vi "dual_color_3D_continuous_scan_with_delay_and_ETL_control.vi"() -> ()   [LabVIEW 2017]
uses:
  <vilib>/DAQmx/write.llb/DAQmx Write (Analog DBL 1Chan 1Samp).vi
  <vilib>/DAQmx/write.llb/DAQmx Write (Analog 1D DBL NChan 1Samp).vi
  <vilib>/DAQmx/write.llb/DAQmx Write (Analog 2D DBL NChan NSamp).vi
  <vilib>/DAQmx/create/channels.llb/DAQmx Create Channel (AO-Voltage-Basic).vi
  <vilib>/DAQmx/miscellaneous.llb/DAQmx Fill In Error Info.vi
  <vilib>/Utility/file.llb/Read Delimited Spreadsheet (DBL).vi
  <vilib>/measure/mascope.llb/Transition Measurements 1 chan.vi
  <vilib>/DAQmx/configure/timing.llb/DAQmx Timing (Sample Clock).vi
  <vilib>/DAQmx/configure/trigger.llb/DAQmx Start Trigger (Digital Edge).vi
  <vilib>/DAQmx/configure/trigger.llb/DAQmx Start Trigger (None).vi
  <vilib>/measure/NI_MAPro.lvlib
panel:
  in  "Listbox 2":i32(listbox)=3
  in  "Listbox":i32(listbox)=1
  in  "ETL voltage offset":dbl(slide) min=-10.0 max=10.0 step=0.05 scale=-10.0..10.0
  out "mirx raw 2":dbl[](array[numeric])
  out "Delay":dbl
  out "Sampling rate":i32
  out "ETL3":waveform(dbl)(graph)
  out "mirror y":waveform(dbl)(graph)
  out "mirror x":waveform(dbl)(graph)
  out "Laser2":waveform(dbl)(graph)
  out "Laser1":waveform(dbl)(graph)
  out "camera":waveform(dbl)(graph)
  out "mirx transition duration":dbl
  out "transition duration":dbl
  out "etl3 timing array":dbl[](array[numeric])
  out "mirror y timing array":dbl[](array[numeric])
  out "mirror x timing array":dbl[](array[numeric])
  out "Laser2 timing array":dbl[](array[numeric])
  out "Laser1 timing array":dbl[](array[numeric])
  out "camera timing array":dbl[](array[numeric])
  out "etl raw":dbl[](array[numeric])
  out "miry raw":dbl[](array[numeric])
  out "mirx raw":dbl[](array[numeric])
  out "Laser2 Intensity":dbl
  out "Laser1 Intensity":dbl
  out "Off Time":dbl
  out "On Time":dbl
  out "Number of slices":dbl
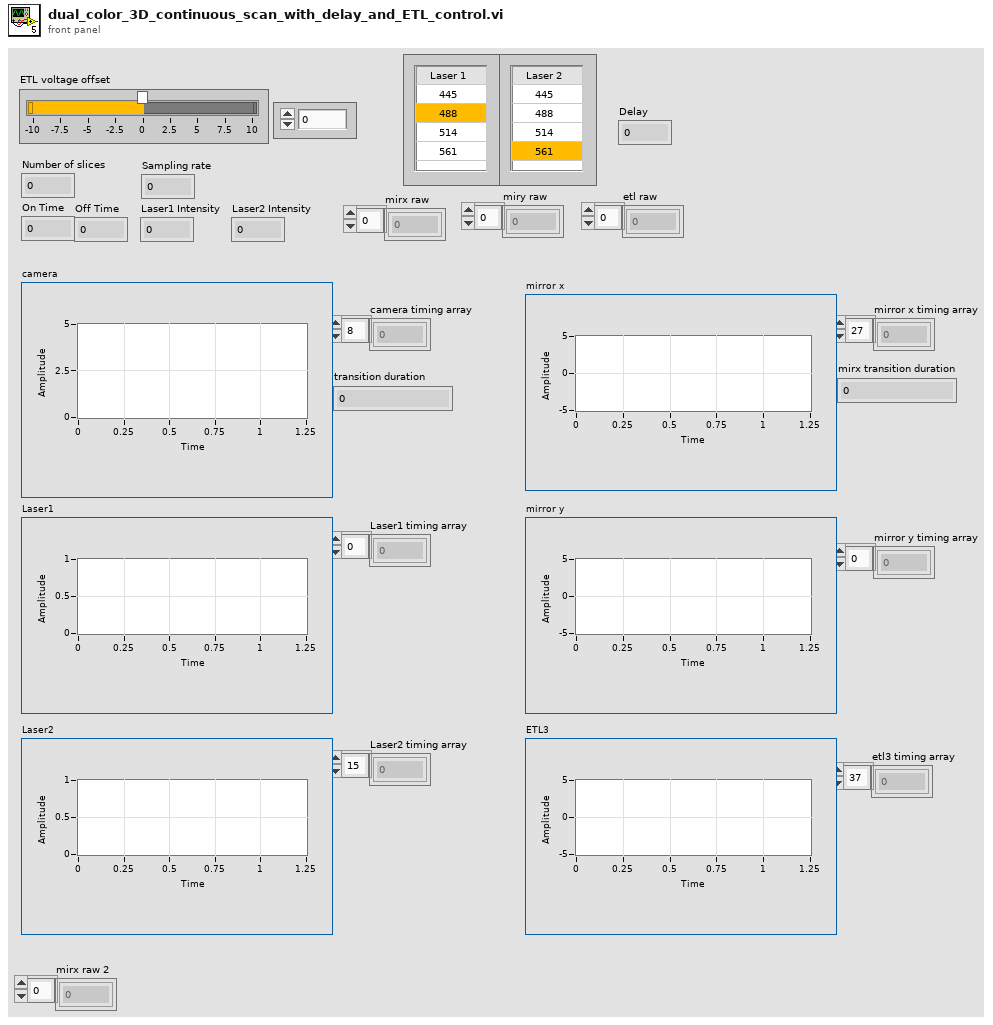
[diagram p1: front panel]
types:
  T1 = enum32{"Invalid", "Standard", "Closed", "Hidden", "Minimized", "Maximized"}
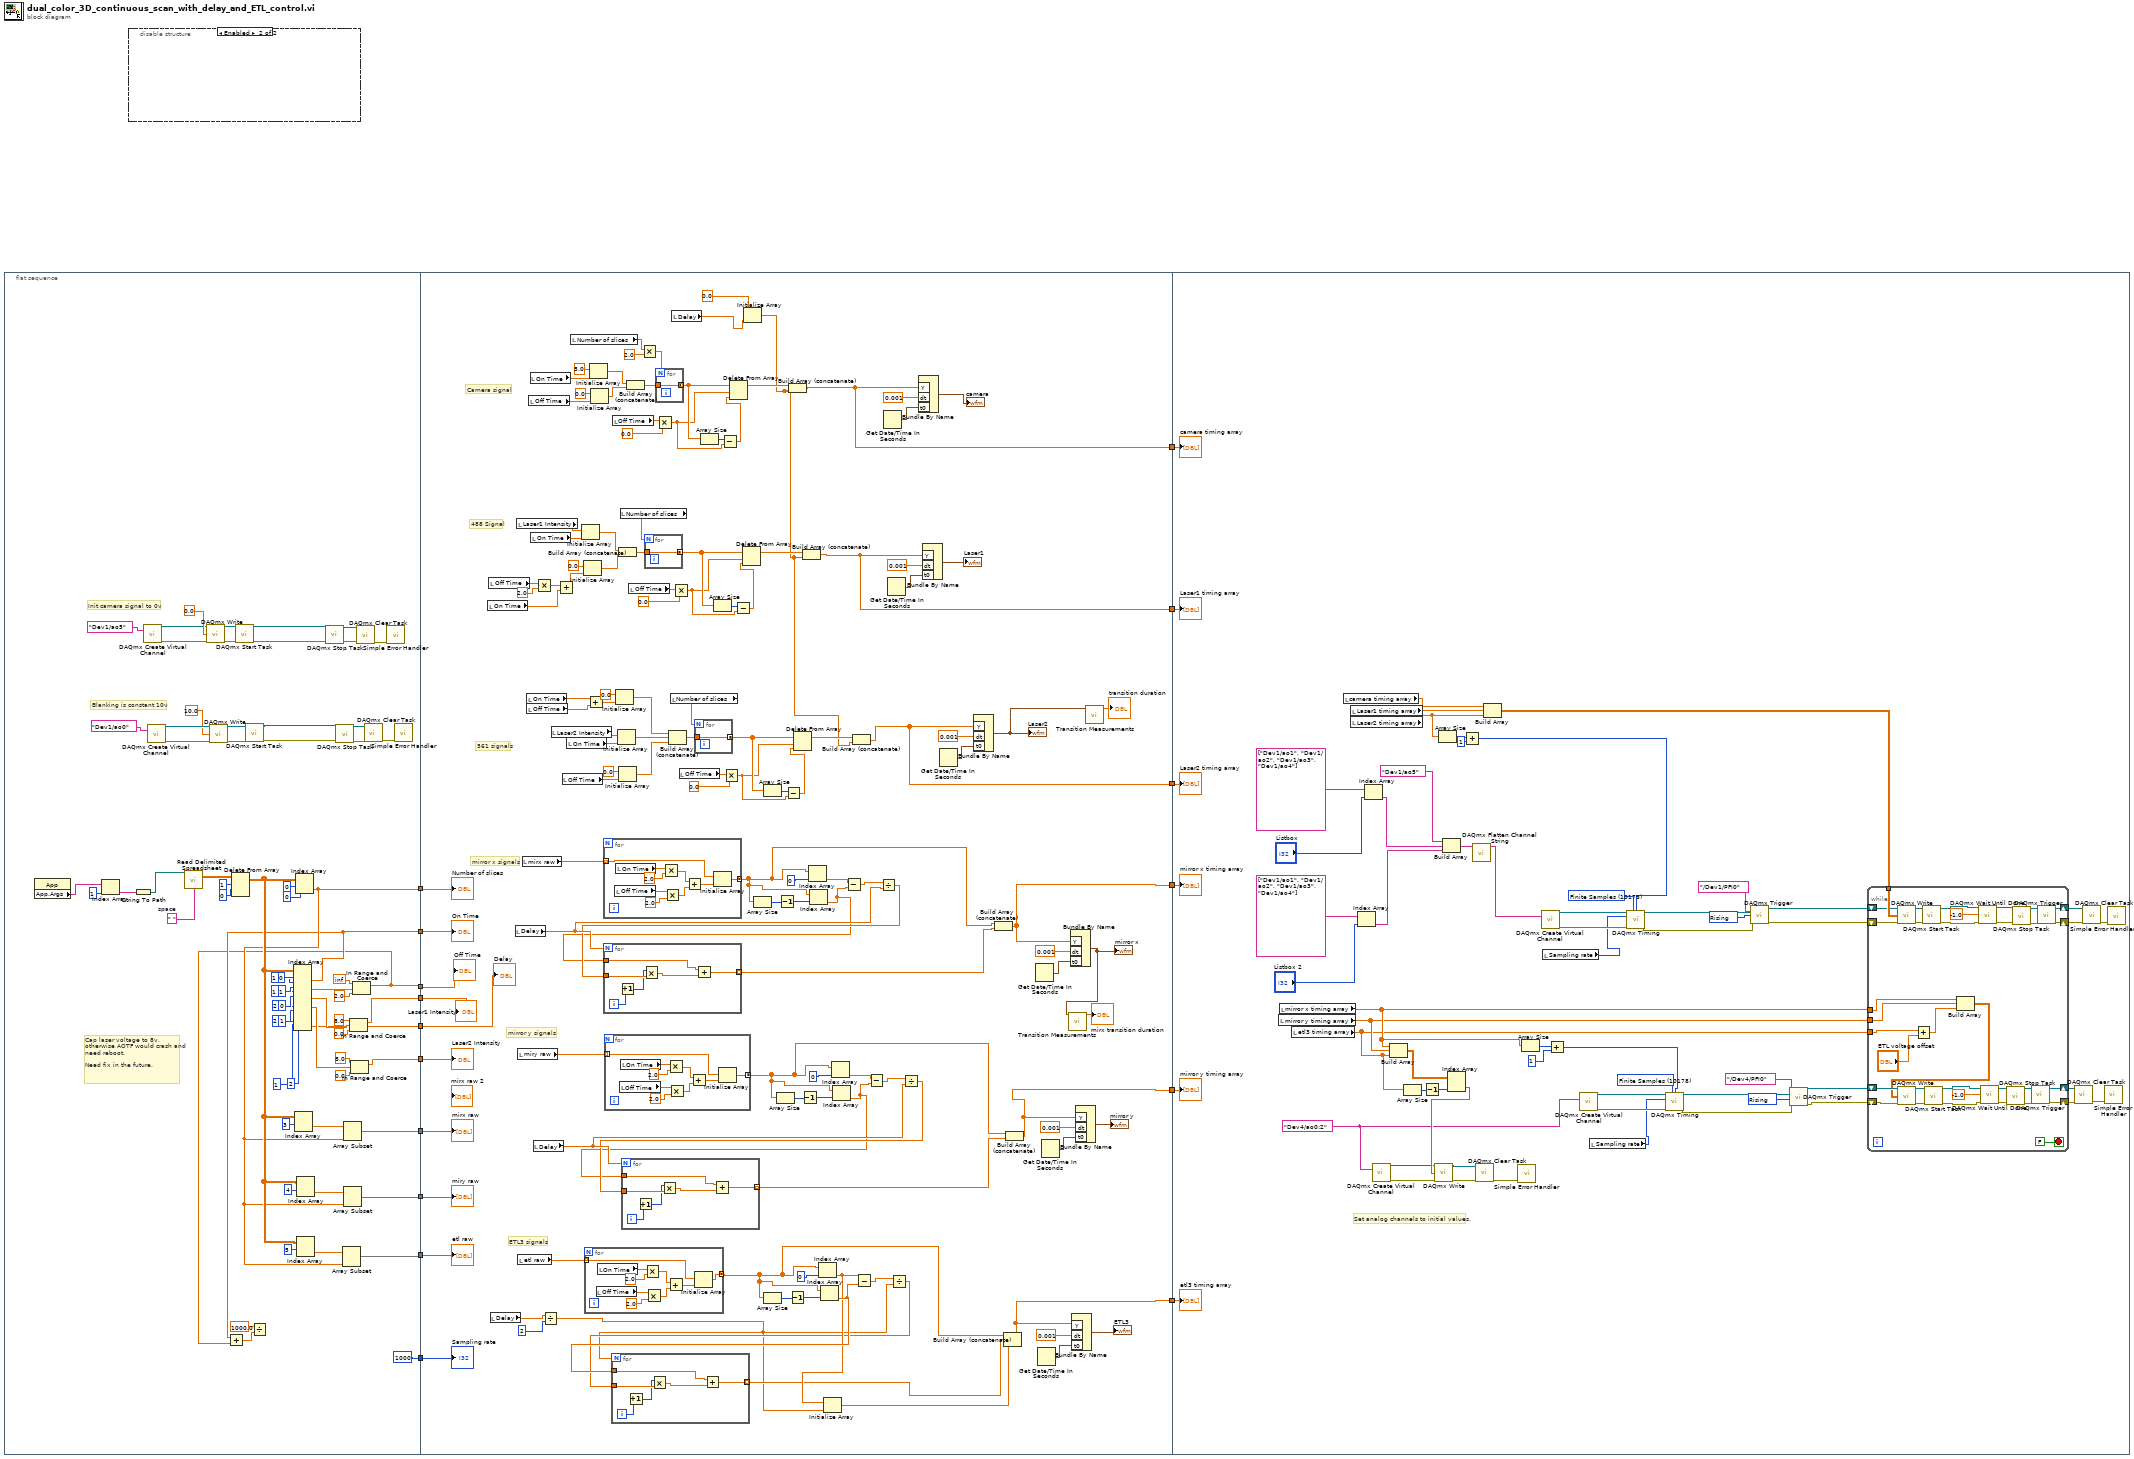
[diagram p0: block diagram]
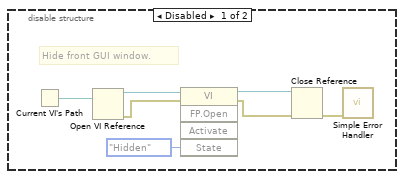
[diagram p2: hidden frame]
diagram:
  n1 = flat-sequence {
    tunnel: [w62] -> w16
    tunnel: [w48] -> w15
    tunnel: [w47] -> w14
    tunnel: [w39] -> w13
    tunnel: [w37] -> w12
    tunnel: [w61] -> w11
    tunnel: [w60] -> w10
    tunnel: [w59] -> w9
    tunnel: [1000] -> w2
    tunnel: [w34] -> w1
    tunnel: w16 -> [w146]
    tunnel: w15 -> [w145]
    tunnel: w14 -> [w144]
    tunnel: w13 -> [w143]
    tunnel: w12 -> [w142]
    tunnel: w11 -> [w141]
    tunnel: w10 -> [w140]
    tunnel: w9 -> [w139]
    tunnel: [w138] -> w8
    tunnel: [w137] -> w7
    tunnel: [w136] -> w6
    tunnel: [w135] -> w5
    tunnel: [w125] -> w4
    tunnel: [w124] -> w3
    tunnel: w2 -> [w126]
    tunnel: w1 -> [w122]
    tunnel: w8 -> [w300]
    tunnel: w7 -> [w299]
    tunnel: w6 -> [w298]
    tunnel: w5 -> [w297]
    tunnel: w4 -> [w296]
    tunnel: w3 -> [w295]
    frame #0 {
      w63 = " "  # space
      # "Init camera signal to 0v"
      # "Cap laser voltage to 8v, otherwise AOTF would crash and need reboot. \n\nNeed fix in the future."
      # "Blanking is constant 10v"
      n2 = property class="App"() -> ("App.Args"=w51:string[])  [unwired: 2 in, 2 out]
      n3 = Index Array(array=w51, index=1) -> (element=w50:string)
      n4 = String To Path(string=w50) -> (path=w49:path)
      n5 = call-poly <vilib>:"DAQmx Create Virtual Channel.vi"("physical channels"=tag "Dev1/ao5") -> ("task out"=w20:refnum<k21>, "error out"=w19:errorcluster)  [unwired: 13 in]
      n6 = call-poly <vilib>:"DAQmx Create Virtual Channel.vi"("physical channels"=tag "Dev1/ao0") -> ("task out"=w57:refnum<k21>, "error out"=w58:errorcluster)  [unwired: 13 in]
      n7 = call-poly <vilib>:"Read Delimited Spreadsheet.vi"("file path (dialog if empty)"=w49, "delimiter (\\t)"=w63) -> ("all rows"=w81:dbl[][])  [unwired: 8 in, 5 out]
      n8 = call-poly <vilib>:"DAQmx Write.vi"("task/channels in"=w20, "data"=0.0, "error in"=w19) -> ("task out"=w27:refnum<k21>, "error out"=w26:errorcluster)  [unwired: 10 in, 1 out]
      n9 = call-poly <vilib>:"DAQmx Write.vi"("task/channels in"=w57, "data"=10.0, "error in"=w58) -> ("task out"=w33:refnum<k21>, "error out"=w32:errorcluster)  [unwired: 10 in, 1 out]
      n10 = Delete From Array(array=w81, length=1, index (row)=0) -> (array with subset deleted=w82:dbl[][])  [unwired: 1 in, 1 out]
      n11 = call <vilib>:"DAQmx Start Task.vi"("task/channels in"=w27, "error in"=w26) -> ("task out"=w18:refnum<k21>, "error out"=w17:errorcluster)  [unwired: 12 in]
      n12 = call <vilib>:"DAQmx Start Task.vi"("task/channels in"=w33, "error in"=w32) -> ("task out"=w29:refnum<k21>, "error out"=w28:errorcluster)  [unwired: 12 in]
      n13 = Index Array(array=w82, index (row) #1=1 ("index (row)"), index (col) #1=0 ("disabled index (col)"), index (row) #2=1 ("index (row)"), index (col) #2=1 ("disabled index (col)"), index (row) #3=2 ("index (row)"), index (col) #3=0 ("disabled index (col)"), index (row) #4=2 ("index (row)"), index (col) #4=1 ("disabled index (col)"), index (row) #6=1 ("index (row)"), index (col) #6=2 ("disabled index (col)")) -> (element #1=w48:dbl, element #2=w86:dbl, element #3=w40:dbl, element #4=w38:dbl, element #6=w34:dbl)  [unwired: 2 in, 1 out]
      n14 = Index Array(array=w82, index (row)=3) -> (element=w83:dbl[])  [unwired: 1 in]
      n15 = Index Array(array=w82, index (row)=0, index (col)=0 ("disabled index (col)")) -> (element=w62:dbl)
      n16 = Index Array(array=w82, index (row)=5) -> (element=w85:dbl[])  [unwired: 1 in]
      n17 = Index Array(array=w82, index (row)=4) -> (element=w84:dbl[])  [unwired: 1 in]
      n18 = call <vilib>:"DAQmx Stop Task.vi"("task/channels in"=w18, "error in"=w17) -> ("task out"=w24:refnum<k21>, "error out"=w25:errorcluster)  [unwired: 12 in]
      n19 = call <vilib>:"DAQmx Stop Task.vi"("task/channels in"=w29, "error in"=w28) -> ("task out"=w31:refnum<k21>, "error out"=w30:errorcluster)  [unwired: 12 in]
      n20 = Array Subset(array=w85, length=w62) -> (w59:dbl[])  [unwired: 1 in]
      n21 = Array Subset(array=w83, length=w62) -> (w61:dbl[])  [unwired: 1 in]
      n22 = Array Subset(array=w84, length=w62) -> (w60:dbl[])  [unwired: 1 in]
      n23 = In Range and Coerce(upper limit=8.0, x=w40, lower limit=0.0) -> (coerced(x)=w39:dbl)  [unwired: 1 out]
      n24 = In Range and Coerce(upper limit=8.0, x=w38, lower limit=0.0) -> (coerced(x)=w37:dbl)  [unwired: 1 out]
      n25 = In Range and Coerce(upper limit=inf, x=w86, lower limit=2.0) -> (coerced(x)=w47:dbl)  [unwired: 1 out]
      n26 = Add(x=w48, y=w47) -> (x+y=w45:dbl)
      n27 = Divide(x=1000.0, y=w45) -> ()  [unwired: 1 out]
      n28 = call <vilib>:"DAQmx Clear Task.vi"("task in"=w24, "error in"=w25) -> ("error out"=w21:errorcluster)  [unwired: 13 in]
      n29 = call <vilib>:"DAQmx Clear Task.vi"("task in"=w31, "error in"=w30) -> ("error out"=w56:errorcluster)  [unwired: 13 in]
      n30 = call <vilib>:"Simple Error Handler.vi"("error in (no error)"=w21) -> ()  [unwired: 4 in, 5 out]
      n31 = call <vilib>:"Simple Error Handler.vi"("error in (no error)"=w56) -> ()  [unwired: 4 in, 5 out]
    }
    frame #1 {
      # "ETL3 signals"
      # "mirror y signals"
      # "mirror x signals"
      # "561 signals"
      # "488 Signal"
      # "Camera signal"
      n32 = local read "On Time"() -> (w193:dbl)
      n33 = local read "Off Time"() -> (w196:dbl)
      n34 = local read "Delay"() -> (w92:dbl)
      n35 = local read "Delay"() -> (w113:dbl)
      n36 = local read "Laser1 Intensity"() -> (w200:dbl)
      n37 = local read "miry raw"() -> (w160:dbl[])
      n38 = local read "etl raw"() -> (w159:dbl[])
      n39 = local read "mirx raw"() -> (w161:dbl[])
      n40 = local read "On Time"() -> (w167:dbl)
      n41 = local read "Off Time"() -> (w178:dbl)
      n42 = local read "Off Time"() -> (w215:dbl)
      n43 = local read "On Time"() -> (w216:dbl)
      n44 = local read "On Time"() -> (w199:dbl)
      n45 = local read "Delay"() -> (w103:dbl)
      n46 = Multiply(x=w196, y=2.0) -> (x*y=w194:dbl)
      n47 = Divide(x=w92, y=2 ("index")) -> (x/y=w87:dbl)
      n48 = local read "Laser2 Intensity"() -> (w181:dbl)
      n49 = Add(x=w194, y=w193) -> (x+y=w192:dbl)
      n50 = local read "Off Time"() -> (w163:dbl)
      n51 = local read "On Time"() -> (w180:dbl)
      n52 = local read "Number of slices"() -> (w208:dbl)
      n53 = Initialize Array(w200, w199) -> (w198:dbl[])
      n54 = Initialize Array(0.0 ("element"), w192) -> (w191:dbl[])
      n55 = for {
        tunnel: w159 -> [w231] mode=indexing
        tunnel: [w230] -> w95 mode=concatenating
        n56 = local read "Off Time"() -> (w236:dbl)
        n57 = local read "On Time"() -> (w234:dbl)
        n58 = Multiply(x=w234, y=2.0) -> (x*y=w235:dbl)
        n59 = Multiply(x=w236, y=2.0) -> (x*y=w237:dbl)
        n60 = Add(x=w235, y=w237) -> (x+y=w238:dbl)
        n61 = Initialize Array(w231, w238) -> (w230:dbl[])
      }
      n62 = Add(x=w167, y=w178) -> (x+y=w177:dbl)
      n63 = Initialize Array(5.0 ("element"), w216) -> (w213:dbl[])
      n64 = Initialize Array(0.0 ("element"), w215) -> (w212:dbl[])
      n65 = for {
        tunnel: w161 -> [w255] mode=indexing
        tunnel: [w254] -> w116 mode=concatenating
        n66 = local read "Off Time"() -> (w260:dbl)
        n67 = local read "On Time"() -> (w262:dbl)
        n68 = Multiply(x=w262, y=2.0) -> (x*y=w261:dbl)
        n69 = Multiply(x=w260, y=2.0) -> (x*y=w259:dbl)
        n70 = Add(x=w261, y=w259) -> (x+y=w258:dbl)
        n71 = Initialize Array(w255, w258) -> (w254:dbl[])
      }
      n72 = for {
        tunnel: w160 -> [w240] mode=indexing
        tunnel: [w239] -> w104 mode=concatenating
        n73 = local read "Off Time"() -> (w245:dbl)
        n74 = local read "On Time"() -> (w243:dbl)
        n75 = Multiply(x=w243, y=2.0) -> (x*y=w244:dbl)
        n76 = Multiply(x=w245, y=2.0) -> (x*y=w246:dbl)
        n77 = Add(x=w244, y=w246) -> (x+y=w247:dbl)
        n78 = Initialize Array(w240, w247) -> (w239:dbl[])
      }
      n79 = local read "Off Time"() -> (w207:dbl)
      n80 = Initialize Array(0.0 ("element"), w177) -> (w166:dbl[])
      n81 = Initialize Array(w181, w180) -> (w165:dbl[])
      n82 = Initialize Array(0.0 ("element"), w163) -> (w162:dbl[])
      n83 = Build Array (concatenate)(w198, w191) -> (w189:dbl[])
      n84 = local read "Number of slices"() -> (w190:dbl)
      n85 = Build Array (concatenate)(w213, w212) -> (w211:dbl[])
      n86 = local read "Off Time"() -> (w185:dbl)
      n87 = Multiply(x=w208, y=2.0) -> (x*y=w210:dbl)
      n88 = for {
        N: w190 -> [_]
        tunnel: w189 -> [w264]
        tunnel: [w264] -> w186 mode=concatenating
      }
      n89 = for {
        N: w210 -> [_]
        tunnel: w211 -> [w265]
        tunnel: [w265] -> w205 mode=concatenating
      }
      n90 = Multiply(x=w207, y=0.0) -> (x*y=w203:dbl)
      n91 = Build Array (concatenate)(w166, w165, w162) -> (w175:dbl[])
      n92 = local read "Number of slices"() -> (w176:dbl)
      n93 = local read "Delay"() -> (w121:dbl)
      n94 = Multiply(x=w185, y=0.0) -> (x*y=w183:dbl)
      n95 = local read "Off Time"() -> (w171:dbl)
      n96 = for {
        N: w176 -> [_]
        tunnel: w175 -> [w263]
        tunnel: [w263] -> w172 mode=concatenating
      }
      n97 = Array Size(array=w205) -> (size(s)=w204:i32)
      n98 = Array Size(array=w186) -> (size(s)=w188:i32)
      n99 = Subtract(x=w204, y=w203) -> (x-y=w202:dbl)
      n100 = Multiply(x=w171, y=0.0) -> (x*y=w169:dbl)
      n101 = Delete From Array(array=w205, length=w203, index=w202) -> (array with subset deleted=w201:dbl[])  [unwired: 1 out]
      n102 = Subtract(x=w188, y=w183) -> (x-y=w187:dbl)
      n103 = Delete From Array(array=w186, length=w183, index=w187) -> (array with subset deleted=w182:dbl[])  [unwired: 1 out]
      n104 = Initialize Array(0.0 ("y"), w121) -> (w120:dbl[])
      n105 = Array Size(array=w116) -> (size(s)=w117:i32)
      n106 = Array Size(array=w172) -> (size(s)=w174:i32)
      n107 = Array Size(array=w95) -> (size(s)=w98:i32)
      n108 = Array Size(array=w104) -> (size(s)=w107:i32)
      n109 = Decrement(x=w117) -> (x-1=w115:i32)
      n110 = Subtract(x=w174, y=w169) -> (x-y=w173:dbl)
      n111 = Build Array (concatenate)(w201, w120) -> (w138:dbl[])
      n112 = Decrement(x=w98) -> (x-1=w97:i32)
      n113 = Delete From Array(array=w172, length=w169, index=w173) -> (array with subset deleted=w168:dbl[])  [unwired: 1 out]
      n114 = Decrement(x=w107) -> (x-1=w106:i32)
      n115 = Build Array (concatenate)(w182, w120) -> (w137:dbl[])
      n116 = Index Array(array=w116, index=0) -> (element=w118:dbl)
      n117 = Index Array(array=w116, index=w115) -> (element=w111:dbl)
      n118 = Index Array(array=w95, index=0) -> (element=w91:dbl)
      n119 = Index Array(array=w95, index=w97) -> (element=w94:dbl)
      n120 = Initialize Array(w91, w87) -> (w88:dbl[])
      n121 = Index Array(array=w104, index=0) -> (element=w108:dbl)
      n122 = Index Array(array=w104, index=w106) -> (element=w101:dbl)
      n123 = Subtract(x=w118, y=w111) -> (x-y=w114:dbl)
      n124 = Build Array (concatenate)(w168, w120) -> (w136:dbl[])
      n125 = Subtract(x=w91, y=w94) -> (x-y=w96:dbl)
      n126 = Subtract(x=w108, y=w101) -> (x-y=w105:dbl)
      n127 = Divide(x=w114, y=w113) -> (x/y=w112:dbl)
      n128 = for {
        N: w113 -> [_]
        tunnel: w112 -> [w253]
        tunnel: w111 -> [w250]
        tunnel: [w248] -> w110 mode=indexing
        i -> [w252]
        n129 = Increment(x=w252) -> (x+1=w251:i32)
        n130 = Multiply(x=w251, y=w253) -> (x*y=w249:dbl)
        n131 = Add(x=w250, y=w249) -> (x+y=w248:dbl)
      }
      n132 = Get Date/Time In Seconds() -> (seconds since 1Jan1904=w153:timestamp)
      n133 = Get Date/Time In Seconds() -> (seconds since 1Jan1904=w151:timestamp)
      n134 = Divide(x=w96, y=w87) -> (x/y=w90:dbl)
      n135 = for {
        N: w87 -> [_]
        tunnel: w90 -> [w223]
        tunnel: w94 -> [w220]
        tunnel: [w218] -> w89 mode=indexing
        i -> [w222]
        n136 = Increment(x=w222) -> (x+1=w221:i32)
        n137 = Multiply(x=w221, y=w223) -> (x*y=w219:dbl)
        n138 = Add(x=w220, y=w219) -> (x+y=w218:dbl)
      }
      n139 = Divide(x=w105, y=w103) -> (x/y=w102:dbl)
      n140 = for {
        N: w103 -> [_]
        tunnel: w102 -> [w229]
        tunnel: w101 -> [w226]
        tunnel: [w224] -> w100 mode=indexing
        i -> [w228]
        n141 = Increment(x=w228) -> (x+1=w227:i32)
        n142 = Multiply(x=w227, y=w229) -> (x*y=w225:dbl)
        n143 = Add(x=w226, y=w225) -> (x+y=w224:dbl)
      }
      n144 = Bundle By Name("Y"=w138, "dt"=0.001, "t0"=w153) -> (→"camera":waveform(dbl))  [unwired: 1 in]
      n145 = Bundle By Name("Y"=w137, "dt"=0.001, "t0"=w151) -> (→"Laser1":waveform(dbl))  [unwired: 1 in]
      n146 = Get Date/Time In Seconds() -> (seconds since 1Jan1904=w155:timestamp)
      n147 = Bundle By Name("Y"=w136, "dt"=0.001, "t0"=w155) -> (w130:waveform(dbl))  [unwired: 1 in]
      "Laser2" <- w130
      n148 = Build Array (concatenate)(w116, w110) -> (w135:dbl[])
      n149 = Build Array (concatenate)(w95, w89, w88) -> (w124:dbl[])
      n150 = Build Array (concatenate)(w104, w100) -> (w125:dbl[])
      n151 = Get Date/Time In Seconds() -> (seconds since 1Jan1904=w157:timestamp)
      n152 = Get Date/Time In Seconds() -> (seconds since 1Jan1904=w147:timestamp)
      n153 = Get Date/Time In Seconds() -> (seconds since 1Jan1904=w149:timestamp)
      n154 = Bundle By Name("Y"=w135, "dt"=0.001, "t0"=w157) -> (w129:waveform(dbl))  [unwired: 1 in]
      "mirror x" <- w129
      n155 = call-poly <vilib>:"Transition Measurements.vi"("signal in"=w129) -> ("transition duration"=→"mirx transition duration":dbl)  [unwired: 5 in, 5 out]
      n156 = Bundle By Name("Y"=w124, "dt"=0.001, "t0"=w147) -> (→"ETL3":waveform(dbl))  [unwired: 1 in]
      n157 = Bundle By Name("Y"=w125, "dt"=0.001, "t0"=w149) -> (→"mirror y":waveform(dbl))  [unwired: 1 in]
      n158 = call-poly <vilib>:"Transition Measurements.vi"("signal in"=w130) -> ("transition duration"=→"transition duration":dbl)  [unwired: 5 in, 5 out]
      "Number of slices" <- w146
      "On Time" <- w145
      "Off Time" <- w144
      "Laser1 Intensity" <- w143
      "Laser2 Intensity" <- w142
      "mirx raw" <- w141
      "miry raw" <- w140
      "etl raw" <- w139
      "Sampling rate" <- w126
      "Delay" <- w122
    }
    frame #2 {
      w306 = 10280 items=["Rising"=10280, "Falling"=10171] ("edge")
      w304 = 10178 items=["Finite Samples"=10178, "Continuous Samples"=10123, "Hardware Timed Single Point"=12522] ("sample mode")
      w305 = tag "Dev4/ao0:2" ("physical channels")
      w302 = 10280 items=["Rising"=10280, "Falling"=10171] ("edge")
      w301 = 10178 items=["Finite Samples"=10178, "Continuous Samples"=10123, "Hardware Timed Single Point"=12522] ("sample mode")
      # "Set analog channels to initial values."
      n159 = local read "mirror y timing array"() -> (w276:dbl[])
      n160 = local read "mirror x timing array"() -> (w277:dbl[])
      n161 = local read "etl3 timing array"() -> (w275:dbl[])
      n162 = local read "camera timing array"() -> (w318:dbl[])
      n163 = local read "Laser1 timing array"() -> (w317:dbl[])
      n164 = local read "Laser2 timing array"() -> (w285:dbl[])
      n165 = Index Array(array=tag[] ["Dev1/ao1", "Dev1/ao2", "Dev1/ao3", "Dev1/ao4"], index="Listbox 2") -> (element=w267:tag)
      n166 = Index Array(array=tag[] ["Dev1/ao1", "Dev1/ao2", "Dev1/ao3", "Dev1/ao4"], index="Listbox") -> (element=w268:tag)
      n167 = call-poly <vilib>:"DAQmx Create Virtual Channel.vi"("physical channels"=w305) -> ("task out"=w313:refnum<k21>, "error out"=w314:errorcluster)  [unwired: 13 in]
      n168 = Build Array(w277, w276, w275) -> (w328:dbl[][])
      n169 = Array Size(array=w275) -> (size(s)=w320:i32)
      n170 = Decrement(x=w320) -> (x-1=w321:i32)
      n171 = Array Size(array=w285) -> (size(s)=w284:i32)
      n172 = Build Array(tag "Dev1/ao5" ("physical channels"), w268, w267) -> (w270:tag[])
      n173 = Index Array(array=w328, index (col)=w321) -> (element=w322:dbl[])  [unwired: 1 in]
      n174 = call-poly <vilib>:"DAQmx Write.vi"("task/channels in"=w313, "data"=w322, "error in"=w314) -> ("task out"=w315:refnum<k21>, "error out"=w316:errorcluster)  [unwired: 10 in, 1 out]
      n175 = Add(x=w284, y=1) -> (x+y=w282:i32)
      n176 = call <vilib>:"DAQmx Flatten Channel String.vi"("names in"=w270) -> ("names out"=w266:string)  [unwired: 13 in, 1 out]
      n177 = call <vilib>:"DAQmx Clear Task.vi"("task in"=w315, "error in"=w316) -> ("error out"=w329:errorcluster)  [unwired: 13 in]
      n178 = Build Array(w318, w317, w285) -> (w319:dbl[][])
      n179 = call <vilib>:"Simple Error Handler.vi"("error in (no error)"=w329) -> ()  [unwired: 4 in, 5 out]
      n180 = Array Size(array=w277) -> (size(s)=w288:i32)
      n181 = call-poly <vilib>:"DAQmx Create Virtual Channel.vi"("physical channels"=w266) -> ("task out"=w309:refnum<k21>, "error out"=w310:errorcluster)  [unwired: 13 in]
      n182 = local read "Sampling rate"() -> (w294:i32)
      n183 = Add(x=w288, y=1) -> (x+y=w286:i32)
      n184 = call-poly <vilib>:"DAQmx Create Virtual Channel.vi"("physical channels"=w305) -> ("task out"=w324:refnum<k21>, "error out"=w325:errorcluster)  [unwired: 13 in]
      n185 = local read "Sampling rate"() -> (w293:i32)
      n186 = call-poly <vilib>:"DAQmx Timing.vi"("task/channels in"=w309, "sample mode"=w301, "samples per channel"=w282, "rate"=w294, "error in"=w310) -> ("task out"=w311:refnum<k21>, "error out"=w312:errorcluster)  [unwired: 9 in]
      n187 = call-poly <vilib>:"DAQmx Timing.vi"("task/channels in"=w324, "sample mode"=w304, "samples per channel"=w286, "rate"=w293, "error in"=w325) -> ("task out"=w326:refnum<k21>, "error out"=w327:errorcluster)  [unwired: 9 in]
      n188 = call-poly <vilib>:"DAQmx Trigger.vi"("task/channels in"=w311, "source"=tag "/Dev1/PFI0", "edge"=w302, "error in"=w312) -> ("task out"=w292:refnum<k21>, "error out"=w291:errorcluster)  [unwired: 10 in]
      n189 = call-poly <vilib>:"DAQmx Trigger.vi"("task/channels in"=w326, "source"=tag "/Dev4/PFI0", "edge"=w306, "error in"=w327) -> ("task out"=w290:refnum<k21>, "error out"=w289:errorcluster)  [unwired: 10 in]
      n190 = while {
        tunnel: w319 -> [w359]
        shift-right: [w338] -> w279
        shift-left: w292 -> [w352]
        shift-right: [w337] -> w278
        shift-left: w291 -> [w351]
        shift-right: [w344] -> w281
        shift-left: w290 -> [w350]
        shift-right: [w343] -> w280
        shift-left: w289 -> [w349]
        tunnel: w277 -> [w334]
        tunnel: w276 -> [w333]
        tunnel: w275 -> [w332]
        stop <- FALSE stop-if-true
        n191 = call-poly <vilib>:"DAQmx Write.vi"("task/channels in"=w352, "data"=w359, "error in"=w351) -> ("task out"=w357:refnum<k21>, "error out"=w358:errorcluster)  [unwired: 10 in, 1 out]
        n192 = Add(x=w332, y="ETL voltage offset") -> (x+y=w330:dbl[])
        n193 = call <vilib>:"DAQmx Start Task.vi"("task/channels in"=w357, "error in"=w358) -> ("task out"=w356:refnum<k21>, "error out"=w355:errorcluster)  [unwired: 12 in]
        n194 = Build Array(w334, w333, w330) -> (w336:dbl[][])
        n195 = call-poly <vilib>:"DAQmx Write.vi"("task/channels in"=w350, "data"=w336, "error in"=w349) -> ("task out"=w362:refnum<k21>, "error out"=w363:errorcluster)  [unwired: 10 in, 1 out]
        n196 = call <vilib>:"DAQmx Start Task.vi"("task/channels in"=w362, "error in"=w363) -> ("task out"=w361:refnum<k21>, "error out"=w360:errorcluster)  [unwired: 12 in]
        n197 = call <vilib>:"DAQmx Wait Until Done.vi"("task/channels in"=w356, "timeout (sec)"=-1.0, "error in"=w355) -> ("task out"=w340:refnum<k21>, "error out"=w339:errorcluster)  [unwired: 11 in]
        n198 = call <vilib>:"DAQmx Wait Until Done.vi"("task/channels in"=w361, "timeout (sec)"=-1.0, "error in"=w360) -> ("task out"=w348:refnum<k21>, "error out"=w347:errorcluster)  [unwired: 11 in]
        n199 = call <vilib>:"DAQmx Stop Task.vi"("task/channels in"=w348, "error in"=w347) -> ("task out"=w346:refnum<k21>, "error out"=w345:errorcluster)  [unwired: 12 in]
        n200 = call <vilib>:"DAQmx Stop Task.vi"("task/channels in"=w340, "error in"=w339) -> ("task out"=w342:refnum<k21>, "error out"=w341:errorcluster)  [unwired: 12 in]
        n201 = call-poly <vilib>:"DAQmx Trigger.vi"("task/channels in"=w346, "error in"=w345) -> ("task out"=w344:refnum<k21>, "error out"=w343:errorcluster)  [unwired: 12 in]
        n202 = call-poly <vilib>:"DAQmx Trigger.vi"("task/channels in"=w342, "error in"=w341) -> ("task out"=w338:refnum<k21>, "error out"=w337:errorcluster)  [unwired: 12 in]
      }
      n203 = call <vilib>:"DAQmx Clear Task.vi"("task in"=w281, "error in"=w280) -> ("error out"=w323:errorcluster)  [unwired: 13 in]
      n204 = call <vilib>:"DAQmx Clear Task.vi"("task in"=w279, "error in"=w278) -> ("error out"=w308:errorcluster)  [unwired: 13 in]
      n205 = call <vilib>:"Simple Error Handler.vi"("error in (no error)"=w323) -> ()  [unwired: 4 in, 5 out]
      n206 = call <vilib>:"Simple Error Handler.vi"("error in (no error)"=w308) -> ()  [unwired: 4 in, 5 out]
      "camera timing array" <- w300
      "Laser1 timing array" <- w299
      "Laser2 timing array" <- w298
      "mirror x timing array" <- w297
      "mirror y timing array" <- w296
      "etl3 timing array" <- w295
    }
  }
  n207 = disable-structure shown="Enabled" {
    frame Disabled {
      # "Hide front GUI window."
      n208 = Current VI's Path() -> (path=w370:path)
      n209 = Open VI Reference(vi path=w370) -> (vi reference=w368:refnum<vi>, error out=w367:errorcluster)  [unwired: 5 in]
      n210 = invoke class="VI" method="FP.Open"(reference=w368, error in=w367, "State"=T1."Hidden") -> (reference out=w366:refnum<vi>, error out=w365:errorcluster)  [unwired: 2 in, 3 out]
      n211 = Close Reference(reference=w366, error in (no error)=w365) -> (error out=w369:errorcluster)
      n212 = call <vilib>:"Simple Error Handler.vi"("error in (no error)"=w369) -> ()  [unwired: 4 in, 5 out]
    }
    frame Enabled {
    }
  }
